vi "DeCoF strip quotation marks.vi"(1 "value":string) -> (0 "trimmed string":string)   [LabVIEW 2013]
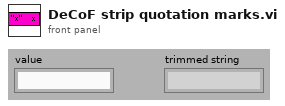
[diagram p1: front panel]
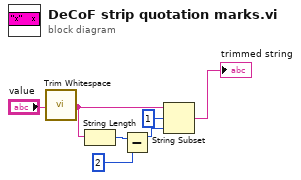
[diagram p0: block diagram]
diagram:
  n1 = call <vilib>:"Trim Whitespace.vi"("string"="value") -> ("trimmed string"=w3:string)  [unwired: 1 in]
  n2 = String Length(string=w3) -> (length=w5:i32)
  n3 = Subtract(x=w5, y=2) -> (x-y=w2:i32)
  n4 = String Subset(string=w3, offset (0)=1, length (rest)=w2) -> (substring=→"trimmed string":string)
